vi "Create New DAQ Data Notifier Name.vi"() -> (0 "Notifier Name":string)   [LabVIEW 2013]
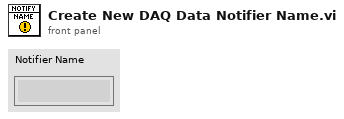
[diagram p1: front panel]
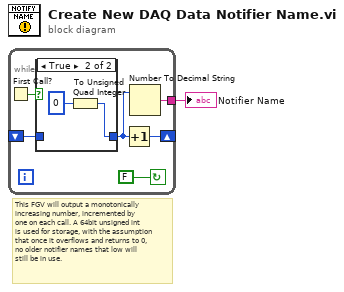
[diagram p0: block diagram]
diagram:
  # "This FGV will output a monotonically\nincreasing number, incremented by\none on each call. A 64bit unsigned int\nis used for storage, with the assumption\nthat once it overflows and returns to 0,\nno older notifier names that low will\nstill be in use."
  n1 = while {
    shift-right: [w5] -> _
    shift-left: _ -> [w6]
    tunnel: [w3] -> w1
    stop <- FALSE continue-if-true
    n2 = First Call?() -> (First Call?: T/F=w7:bool)
    n3 = case shown="True" w7 {
      tunnel: [w8 w9] -> w4
      tunnel: w6 -> [w8 _]
      frame False {
      }
      frame True {
        n4 = To Unsigned Quad Integer(1:0) -> (0:w9:u64)
      }
    }
    n5 = Increment(x=w4) -> (x+1=w5:u64)
    n6 = Number To Decimal String(number=w4) -> (decimal integer string=w3:string)  [unwired: 1 in]
  }
  "Notifier Name" <- w1
